vi "Actor Core.vi"(8 "error in":errorcluster, 11 "Form Model in":refnum<class "Form Model.lvclass">) -> (0 "error out":errorcluster, 3 "Actor out":refnum<class "Actor.lvclass">)   [LabVIEW 2020, in "Form Model.lvlib" / "Form Model.lvclass"]
doc: "(<B>Filename</B>: Actor Framework.lvlib:Actor.lvclass:Actor Core.vi)\n\nReceives messages to the actor, reacts to them, and initiates any error handling that may shut the actor down.\n\nDescendant classes may override this VI to append parallel tasks for the actor to complete while it handles messages. Overrides use the Call Parent Class Method node."
uses:
  Form Model.lvclass
  C:/Program Files (x86)/National Instruments/LabVIEW 2020/vi.lib/ActorFramework/Actor/Actor.lvclass
  <vilib>/ActorFramework/Actor/Actor.lvclass
  Form Controller/Panel Form Controller.lvclass
  C:/Program Files (x86)/National Instruments/LabVIEW 2020/vi.lib/MGI/Panel Manager/Panel Actor/Panel Actor/Panel Actor.lvclass
  Form Model.lvclass/Form Model.ctl
  Form Configuration/Form Configuration.lvclass/Form Configuration.ctl
  Form Controller/Panel Form Controller.lvclass/Panel Form Controller.ctl
  <vilib>/MGI/Panel Manager/Panel Actor/Panel Actor/Launch as Nested Actor.vi
  source/Database/Database.lvclass
  <vilib>/MGI/Panel Manager/Panel/Panel/Panel.lvclass
  <vilib>/MGI/Monitored Actor/Monitored Actor/Monitored Actor/Monitored Actor.lvclass
  Form Configuration/Form Configuration.lvclass
  <vilib>/MGI/Panel Manager/Panel Actor/Panel Actor/Panel Actor.lvclass
  C:/Program Files (x86)/National Instruments/LabVIEW 2020/vi.lib/MGI/Monitored Actor/Monitored Actor/Monitored Actor/Monitored Actor.lvclass
  C:/Users/User/Desktop/Raman Program/Database OOP/forms AF/Form Controller/Panel Form Controller.lvclass
  C:/Users/User/Desktop/Raman Program/Database OOP/forms AF/Form Model/Form Model.lvclass
  C:/Users/User/Desktop/Raman Program/Database OOP/forms AF/Form Model Messages/Form Model Messages.lvclass
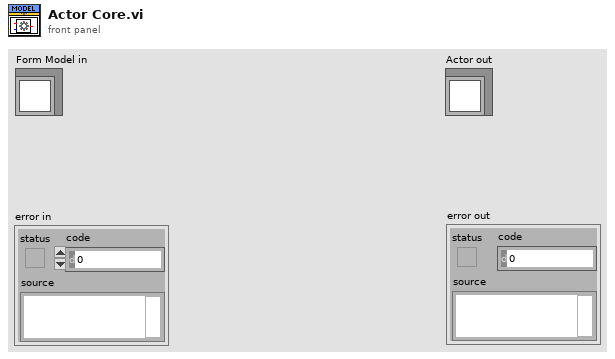
[diagram p1: front panel]
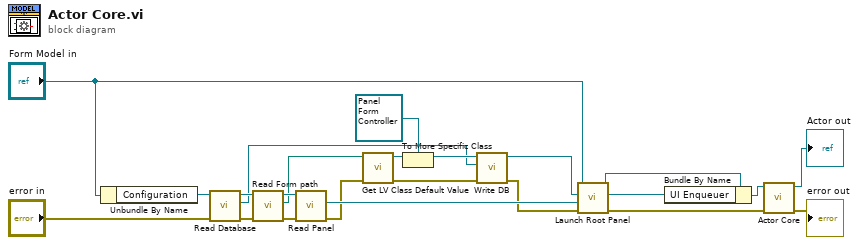
[diagram p0: block diagram]
diagram:
  n1 = Unbundle By Name("Form Model in") -> ("Configuration"=w5:refnum<class "Form Configuration.lvclass">)
  n2 = call "Read Database.vi"("error in (no error)"="error in", "Form Configuration in"=w5) -> ("error out"=w2:errorcluster, "Database.lvclass"=w1:refnum<class "Database.lvclass">, "Form Configuration out"=w4:refnum<class "Form Configuration.lvclass">)  [unwired: 7 in]
  n3 = call "Read Form path.vi"("error in (no error)"=w2, "Form Configuration in"=w4) -> ("error out"=w14:errorcluster, "Form path"=w18:path, "Form Configuration out"=w19:refnum<class "Form Configuration.lvclass">)  [unwired: 7 in]
  n4 = call "Read Panel.vi"("error in (no error)"=w14, "Form Configuration in"=w19) -> ("error out"=w13:errorcluster, "Panel.lvlib:Panel.lvclass"=w20:refnum<class "Panel.lvclass">)  [unwired: 7 in, 1 out]
  n5 = call <vilib>:"Get LV Class Default Value.vi"("error in (no error)"=w13, "class path"=w18) -> ("error out"=w12:errorcluster, "object"=w17:refnum<class>)  [unwired: 8 in]
  n6 = To More Specific Class(target class=refnum<class "Panel Form Controller.lvclass"> refnum ("Panel Form Controller.lvlib:Panel Form Controller.lvclass"), reference=w17) -> (specific class reference=w15:refnum<class "Panel Form Controller.lvclass">)  [unwired: 1 in, 1 out]
  n7 = call "Write DB.vi"("error in (no error)"=w12, "Database.lvclass"=w1, "Panel Form Controller in"=w15) -> ("error out"=w10:errorcluster, "Panel Form Controller out"=w11:refnum<class "Panel Form Controller.lvclass">)  [unwired: 7 in]
  n8 = call-poly <vilib>:"Launch Root Panel.vi"("Error In"=w10, "Panel"=w20, "Panel Actor in"=w11, "Caller Actor in"="Form Model in") -> ("Error Out"=w6:errorcluster, "Actor's Enqueuer"=w8:refnum<class "Message Enqueuer.lvclass">, "Caller Actor out"=w9:refnum<class "Form Model.lvclass">)  [unwired: 5 in]
  n9 = Bundle By Name(cluster=w9, "UI Enqueuer"=w8) -> (w7:refnum<class "Form Model.lvclass">)
  n10 = call-parent "Actor Core.vi"("error in"=w6, "Actor in"=w7) -> ("error out"=→"error out":errorcluster, "Actor out"=→"Actor out":refnum<class "Actor.lvclass">)  [unwired: 8 in]
